vi "StatisticForVelocities1.vi"(6 "Path Vel (1D)":dbl[](array[numeric]), 7 "Intervals":i32=10, 8 "Instant Vel (1D)":dbl[](array[numeric])) -> (0 "StD Path":dbl format="%0.2f", 1 "mean Path Vel":dbl format="%0.2f", 2 "All Path Vel":T1(graph), 3 "All Instant Vel":T1(graph), 4 "mean Instant Vel":dbl format="%0.2f", 5 "StD Instant":dbl format="%0.2f")   [LabVIEW 2013]
uses:
  <vilib>/Analysis/NI_AALBase.lvlib
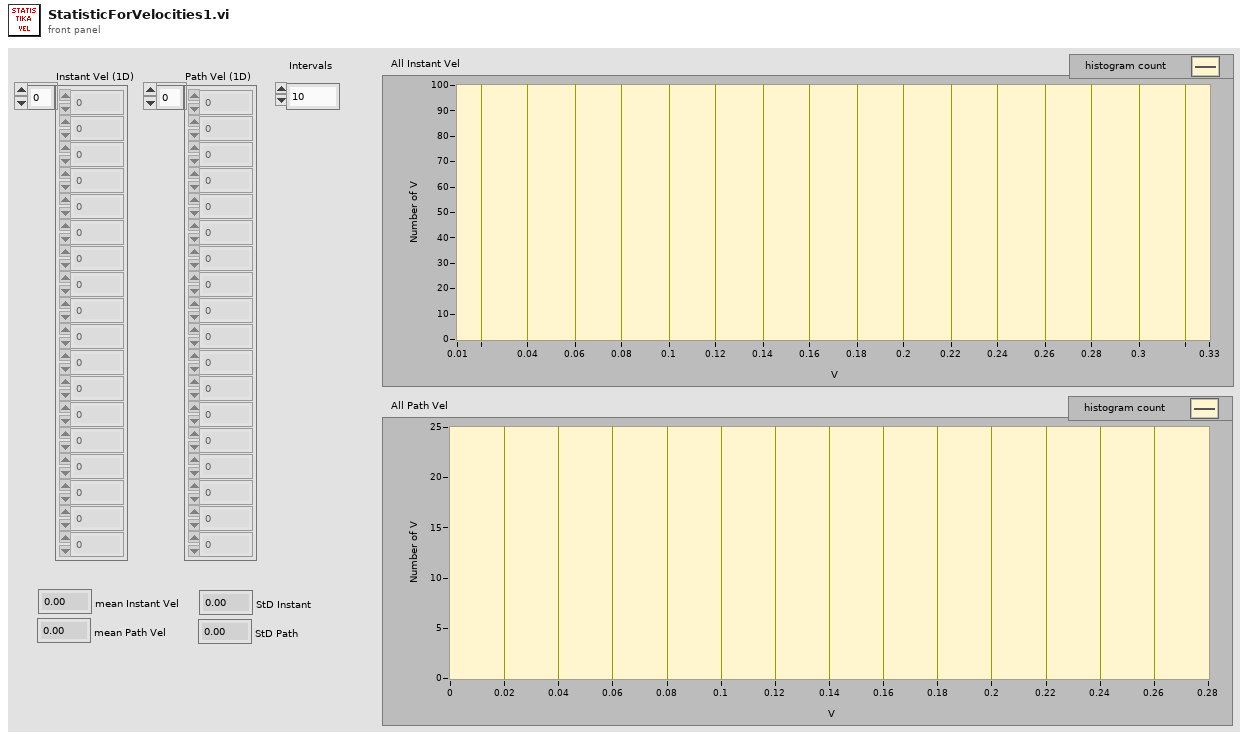
[diagram p1: front panel]
types:
  T1 = cluster{"X Values":dbl[], "Histogram: h(x)":i32[]}
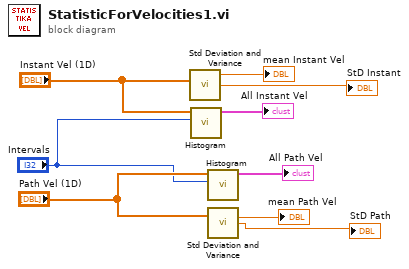
[diagram p0: block diagram]
diagram:
  n1 = call <vilib>:"Std Deviation and Variance.vi"("X"="Instant Vel (1D)") -> ("mean"=→"mean Instant Vel":dbl, "standard deviation"=→"StD Instant":dbl)  [unwired: 1 in, 1 out]
  n2 = call <vilib>:"Histogram.vi"("intervals"="Intervals", "X"="Instant Vel (1D)") -> ("Histogram Graph"=→"All Instant Vel":T1)  [unwired: 6 in, 3 out]
  n3 = call <vilib>:"Histogram.vi"("intervals"="Intervals", "X"="Path Vel (1D)") -> ("Histogram Graph"=→"All Path Vel":T1)  [unwired: 6 in, 3 out]
  n4 = call <vilib>:"Std Deviation and Variance.vi"("X"="Path Vel (1D)") -> ("mean"=→"mean Path Vel":dbl, "standard deviation"=→"StD Path":dbl)  [unwired: 1 in, 1 out]
